vi "copy file.vi"(8 "error in (no error)":errorcluster, 10 "目标路径（使用对话框）":path, 11 "源路径":path) -> (0 "error out":errorcluster)   [LabVIEW 2016, in "数据传输系统-04.lvlib" / "update.lvlib"]
uses:
  update.lvlib
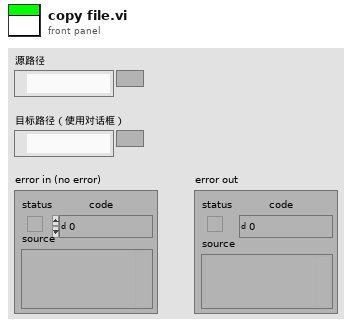
[diagram p1: front panel]
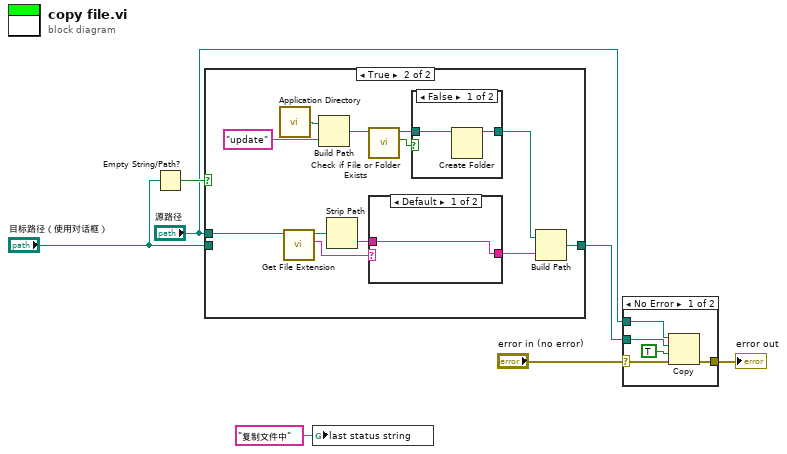
[diagram p0: block diagram]
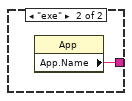
[diagram p3: hidden frame]
diagram:
  n1 = Empty String/Path?(string/path="目标路径（使用对话框）") -> (empty?=w5:bool)
  n2 = case shown="True" w5 {
    tunnel: [w8 w10] -> w2
    tunnel: "目标路径（使用对话框）" -> [w8 _]
    tunnel: "源路径" -> [_ w15]
    frame False {
    }
    frame True {
      n3 = call <vilib>:"Application Directory.vi"() -> ("Application Directory"=w19:path)
      n4 = call <vilib>:"Get File Extension.vi"("file"=w15) -> ("lowercase file extension"=w14:string, "dup file"=w13:path)  [unwired: 6 in, 3 out]
      n5 = Build Path(base path=w19, name or relative path="update" ("名称或相对路径")) -> (appended path=w20:path)
      n6 = Strip Path(path=w13) -> (name=w9:string)  [unwired: 1 out]
      n7 = call <vilib>:"Check if File or Folder Exists.vi"("path"=w20) -> ("file or folder exists?"=w16:bool, "dup path"=w17:path)  [unwired: 8 in, 1 out]
      n8 = case shown="Default" w14 {
        tunnel: [w21 w22] -> w11
        tunnel: w9 -> [w21 _]
        frame Default {
        }
        frame "exe" {
          n9 = property class="App"() -> ("App.Name"=w22:string)  [unwired: 2 in, 2 out]
        }
      }
      n10 = case shown="False" w16 {
        tunnel: w17 -> [w24 w25]
        tunnel: [w23 w25] -> w12
        frame False {
          n11 = Create Folder(path (use dialog)=w24) -> (created path=w23:path)  [unwired: 2 in, 2 out]
        }
        frame True {
        }
      }
      n12 = Build Path(base path=w12, name or relative path=w11) -> (appended path=w10:path)
    }
  }
  n13 = global write "更新全局变量.vi" "last status string"("复制文件中" ("last status string")) -> ()
  n14 = case shown="No Error" "error in (no error)" {
    selector: "error in (no error)" -> [w26 w31]
    tunnel: [w29 w31] -> w6
    tunnel: "源路径" -> [w28 _]
    tunnel: w2 -> [w27 _]
    frame No Error {
      n15 = Copy(8:w26, 9:TRUE ("覆盖(F)"), 10:w27, 11:w28) -> (0:w29:errorcluster)  [unwired: 1 in, 2 out]
    }
    frame Error {
    }
  }
  "error out" <- w6
